vi "ASIA Reserve Pump.vi"(8 "error in (no error)":errorcluster, 11 "ASIA Pump # In":i32) -> (0 "error out":errorcluster, 3 "ASIA Pump # Out":i32)   [LabVIEW 2018, in "ASIA Pump.lvlib"]
uses:
  ASIA Pump.lvlib
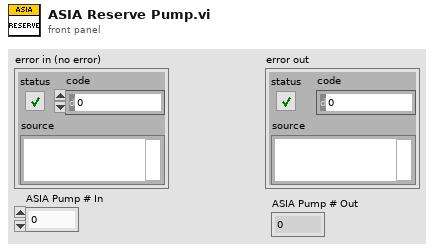
[diagram p1: front panel]
types:
  T1 = cluster{"Busy":bool, "PumpCnt":dbl, "RemoteEntered":bool, "OverpressureSet":bool}[]
  T2 = cluster{"Busy":bool, "PumpCnt":dbl, "RemoteEntered":bool, "OverpressureSet":bool}
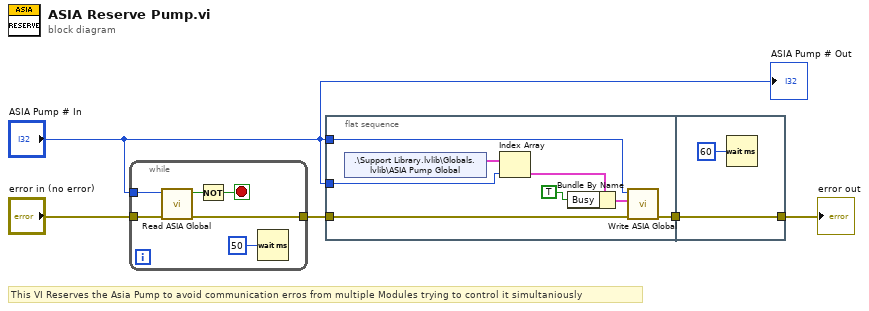
[diagram p0: block diagram]
diagram:
  # "This VI Reserves the Asia Pump to avoid communication erros from multiple Modules trying to control it simultaniously"
  n1 = while {
    tunnel: "ASIA Pump # In" -> [w11]
    tunnel: [w8] -> w5
    tunnel: "error in (no error)" -> [w7]
    stop <- w9 stop-if-true
    n2 = call "Read ASIA Global.vi"("error in (no error)"=w7, "Pump Number"=w11) -> ("error out"=w8:errorcluster, "Busy"=w10:bool)  [unwired: 8 in]
    n3 = Not(x=w10) -> (.not. x?=w9:bool)
    n4 = Wait (ms)(milliseconds to wait=u32 50) -> ()  [unwired: 1 out]
  }
  n5 = flat-sequence {
    tunnel: w5 -> [w19]
    tunnel: "ASIA Pump # In" -> [w17]
    tunnel: [w18] -> w2
    tunnel: "ASIA Pump # In" -> [w15]
    tunnel: [w21] -> w3
    tunnel: w2 -> [w21]
    frame #0 {
      n6 = shared-variable ".\\Support Library.lvlib\\Globals.lvlib\\ASIA Pump Global"() -> (w16:T1)  [unwired: 1 in, 1 out]
      n7 = Index Array(array=w16, index=w15) -> (element=w12:T2)
      n8 = Bundle By Name(cluster=w12, "Busy"=TRUE) -> (w13:T2)
      n9 = call "Write ASIA Global.vi"("error in (no error)"=w19, "ASIA Global"=w13, "Pump Number In"=w17) -> ("error out"=w18:errorcluster)  [unwired: 7 in, 1 out]
    }
    frame #1 {
      n10 = Wait (ms)(milliseconds to wait=u32 60) -> ()  [unwired: 1 out]
    }
  }
  "error out" <- w3
  "ASIA Pump # Out" <- "ASIA Pump # In"
